vi "fgv buffer image references - measure tool.vi"(0 "Image Reference IN":T4, 1 "Actions":T1, 2 "Path":path, 5 "Imaging Parameters":T2, 9 "Calibration Parameters":T3, 11 "error in (no error)":errorcluster, 12 "index(s)":i32[](array[numeric]), 13 "element":string) -> (3 "Imag ref. name":string[](array[string]), 4 "Image Array":T4[](array[typedef]), 6 "LB data":string[][](array[string]), 8 "Imaging Parameters":T2[](array[typedef]), 10 "Calibration Parameters":T3[](array[typedef]), 14 "LB data full":string[][](array[string]), 15 "error out":errorcluster)   [LabVIEW 2020]
uses:
  <vilib>/vision/Image Controls.llb/IMAQ Image.ctl
  ToolBox/TypeDefs/Current Calibration Parameters.ctl
  ToolBox/TypeDefs/Current Imaging Parameters.ctl
  ToolBox/TypeDefs/data and image buffer fgv actions - measure tool.ctl
  138bf972-3e2c-4b9c-869a-8880fb0fa013.vi
  34bb193f-b545-427e-b1e4-c07e80b324ef.vi
  f5771faa-6821-441f-a328-0f121c78e6d9.vi
  d3480d6e-a209-486d-a997-ed0cab6325bc.vi
  <vilib>/Analysis/1siggen.llb/Ramp Pattern by Samples.vi
  <vilib>/Analysis/NI_AALBase.lvlib
panel:
  out "Sr No.":i32[](array[numeric])
  # "Note elements and index(s) are multi-use"
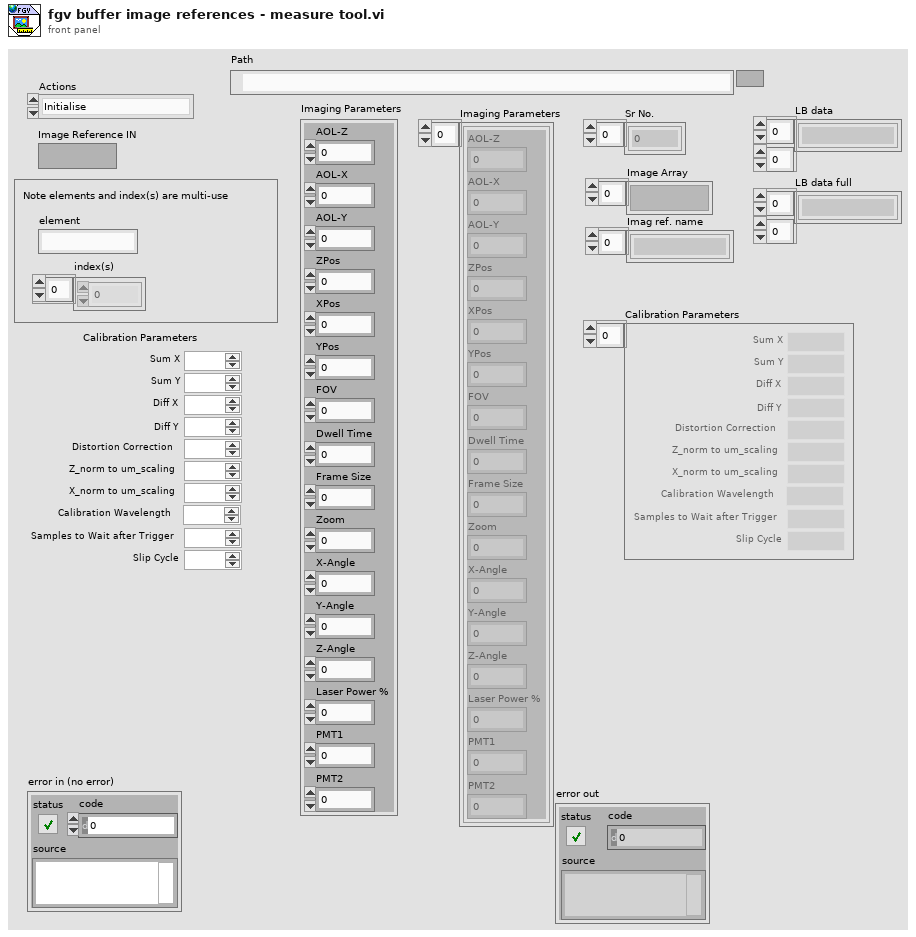
[diagram p1: front panel]
types:
  T1 = typedef "data and image buffer fgv actions - measure tool.ctl" = enum16{"Initialise", "Load Data from file", "Add Image to buffer", "Read Image buffer", "Edit specific data", "Delete selected image", "Clear all images"}
  T2 = typedef "Current Imaging Parameters.ctl" = cluster{"AOL-Z":dbl, "AOL-X":dbl, "AOL-Y":dbl, "ZPos":dbl, "XPos":dbl, "YPos":dbl, "FOV":dbl, "Dwell Time":dbl, "Frame Size":dbl, "Zoom":dbl, "X-Angle":dbl, "Y-Angle":dbl, "Z-Angle":dbl, "Laser Power %":dbl, "PMT1":dbl, "PMT2":dbl}
  T3 = typedef "Current Calibration Parameters.ctl" = cluster{"Sum X":dbl, "Sum Y":dbl, "Diff X":dbl, "Diff Y":dbl, "Distortion Correction":dbl, "Z_norm to um_scaling":dbl, "X_norm to um_scaling":dbl, "Samples to Wait after Trigger":dbl, "Slip Cycle":dbl, "Calibration Wavelength":dbl}
  T4 = typedef "IMAQ Image.ctl" = refnum<image>
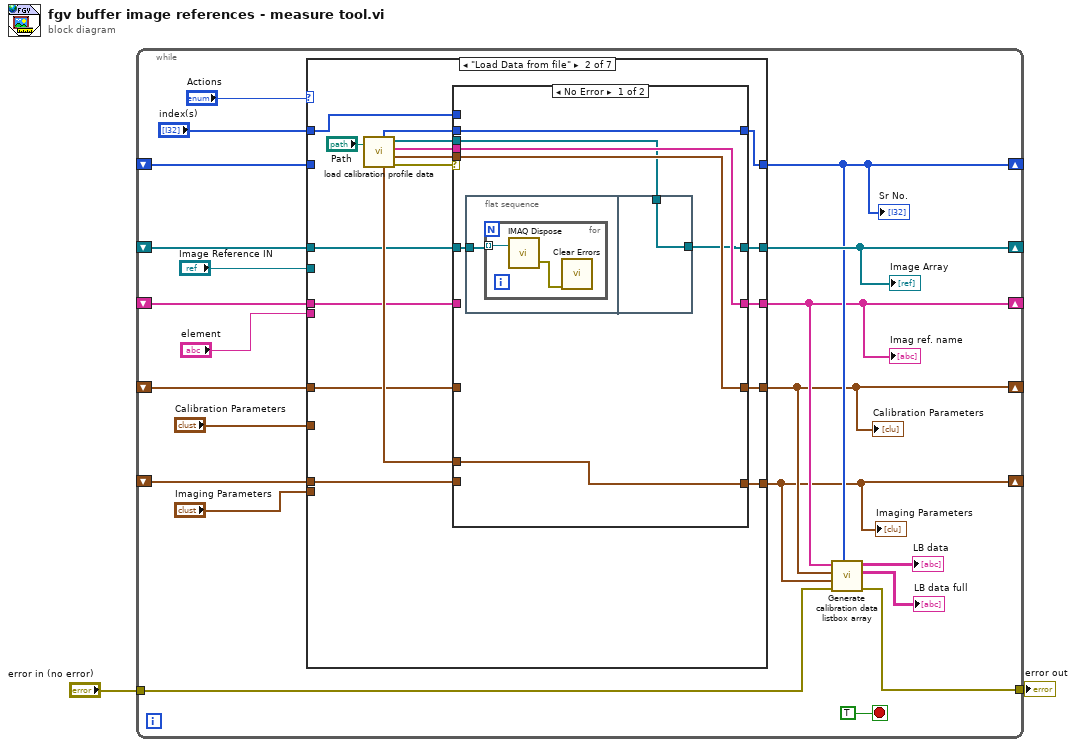
[diagram p0: block diagram]
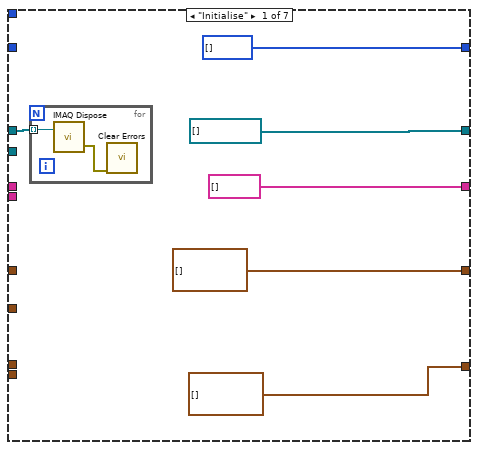
[diagram p2: hidden frame]
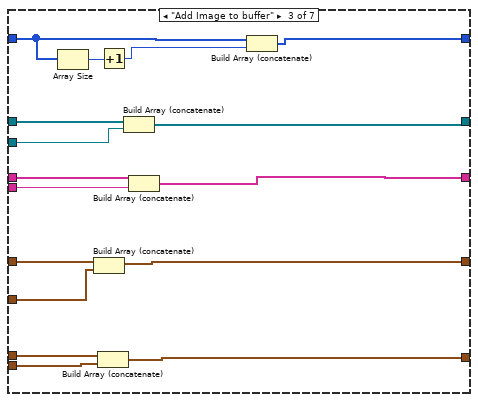
[diagram p4: hidden frame]
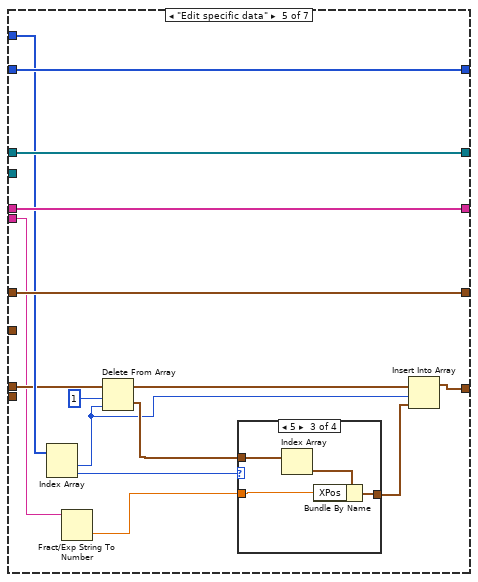
[diagram p6: hidden frame]
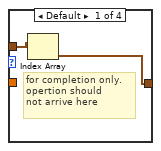
[diagram p7: hidden frame]
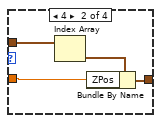
[diagram p8: hidden frame]
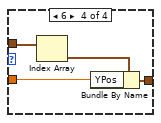
[diagram p9: hidden frame]
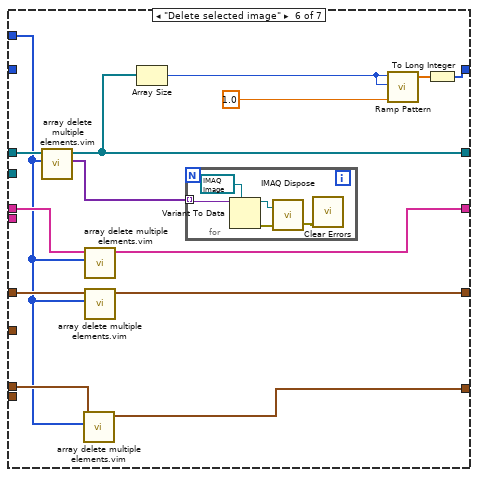
[diagram p10: hidden frame]
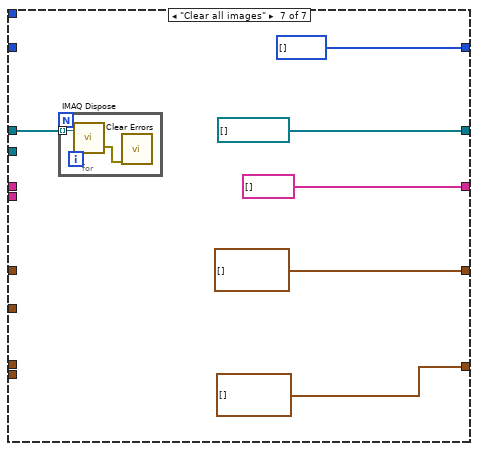
[diagram p11: hidden frame]
diagram:
  n1 = while {
    shift-right: [w22] -> _
    shift-left: _ -> [w21]
    tunnel: "error in (no error)" -> [w7]
    tunnel: [w6] -> w1
    shift-right: [w9] -> _
    shift-left: _ -> [w20]
    shift-right: [w8] -> _
    shift-left: _ -> [w18]
    shift-right: [w10] -> _
    shift-left: _ -> [w16]
    shift-right: [w11] -> _
    shift-left: _ -> [w12]
    stop <- TRUE stop-if-true
    n2 = case shown="\"Load Data from file\"" "Actions" {
      tunnel: [T4[] [] ("RedImageArray") w45 w79 w85 w99 w120 T4[] [] ("RedImageArray")] -> w22
      tunnel: w21 -> [w28 w35 w80 w85 w99 w124 w139]
      tunnel: "index(s)" -> [_ w37 _ _ w96 w116 _]
      tunnel: [T3[] [] w41 w65 w84 w97 w127 T3[] []] -> w9
      tunnel: w20 -> [_ w33 w78 w84 w97 w128 _]
      tunnel: "Calibration Parameters" -> [_ _ w77 _ _ _ _]
      tunnel: [T2[] [] w38 w67 w83 w86 w125 T2[] []] -> w8
      tunnel: w18 -> [_ w32 w76 w83 w95 w126 _]
      tunnel: "Imaging Parameters" -> [_ _ w75 _ _ _ _]
      tunnel: [string[] [] w43 w66 w81 w98 w115 string[] []] -> w10
      tunnel: w16 -> [_ w34 w74 w81 w98 w117 _]
      tunnel: "element" -> [_ _ w73 _ w91 _ _]
      tunnel: [i32[] [] w36 w68 w82 w100 w118 i32[] []] -> w11
      tunnel: "Image Reference IN" -> [_ _ w72 _ _ _ _]
      tunnel: w12 -> [_ _ w70 w82 w100 _ _]
      frame "Initialise" {
        n3 = for {
          tunnel: w28 -> [w31] mode=indexing
          n4 = call "IMAQ Dispose"("Image"=w31) -> ("error out"=w30:errorcluster)  [unwired: 5 in]
          n5 = call <vilib>:"Clear Errors.vi"("error in (no error)"=w30) -> ()  [unwired: 5 in, 2 out]
        }
      }
      frame "Load Data from file" {
        n6 = call "load calibration profile data.vi"("Path"="Path") -> ("error out"=w47:errorcluster, "Calibration params"=w40:T3[], "Image names"=w42:string[], "Image Array refs"=w44:T4[], "Scanning params"=w39:T2[], "Sr No."=w46:i32[])  [unwired: 5 in]
        n7 = case shown="No Error" w47 {
          tunnel: [w55 w64] -> w36
          tunnel: w46 -> [w55 _]
          tunnel: [w50 w63] -> w45
          tunnel: w44 -> [w49 _]
          tunnel: [w54 w62] -> w43
          tunnel: w42 -> [w54 _]
          tunnel: [w53 w61] -> w41
          tunnel: w40 -> [w53 _]
          tunnel: w39 -> [w52 _]
          tunnel: [w52 w60] -> w38
          tunnel: w37 -> [_ w64]
          tunnel: w35 -> [w51 w63]
          tunnel: w34 -> [_ w62]
          tunnel: w33 -> [_ w61]
          tunnel: w32 -> [_ w60]
          frame No Error {
            n8 = flat-sequence {
              tunnel: w51 -> [w56]
              tunnel: [w59] -> w50
              tunnel: w49 -> [w59]
              frame #0 {
                n9 = for {
                  tunnel: w56 -> [w58] mode=indexing
                  n10 = call "IMAQ Dispose"("Image"=w58) -> ("error out"=w57:errorcluster)  [unwired: 5 in]
                  n11 = call <vilib>:"Clear Errors.vi"("error in (no error)"=w57) -> ()  [unwired: 5 in, 2 out]
                }
              }
              frame #1 {
              }
            }
          }
          frame Error {
          }
        }
      }
      frame "Add Image to buffer" {
        n12 = Array Size(array=w70) -> (size(s)=w71:i32)
        n13 = Build Array (concatenate)(w78, w77) -> (w65:T3[])
        n14 = Build Array (concatenate)(w76, w75) -> (w67:T2[])
        n15 = Increment(x=w71) -> (x+1=w69:i32)
        n16 = Build Array (concatenate)(w80, w72) -> (w79:T4[])
        n17 = Build Array (concatenate)(w74, w73) -> (w66:string[])
        n18 = Build Array (concatenate)(w70, w69) -> (w68:i32[])
      }
      frame "Read Image buffer" {
      }
      frame "Edit specific data" {
        n19 = Index Array(array=w96) -> (element #1=w89:i32, element #2=w93:i32)  [unwired: 2 in]
        n20 = Fract/Exp String To Number(string=w91) -> (number=w90:dbl)  [unwired: 3 in, 1 out]
        n21 = Delete From Array(array=w95, length=1, index=w89) -> (deleted portion=w92:T2[], array with subset deleted=w88:T2[])
        n22 = case shown="5" w93 {
          tunnel: w92 -> [w102 w105 w109 w114]
          tunnel: w90 -> [_ w104 w108 w112]
          tunnel: [w101 w103 w107 w111] -> w87
          frame Default {
            # "for completion only.\nopertion should \nnot arrive here"
            n23 = Index Array(array=w102) -> (element=w101:T2)  [unwired: 1 in]
          }
          frame 4 {
            n24 = Index Array(array=w105) -> (element=w106:T2)  [unwired: 1 in]
            n25 = Bundle By Name(cluster=w106, "ZPos"=w104) -> (w103:T2)
          }
          frame 5 {
            n26 = Index Array(array=w109) -> (element=w110:T2)  [unwired: 1 in]
            n27 = Bundle By Name(cluster=w110, "XPos"=w108) -> (w107:T2)
          }
          frame 6 {
            n28 = Index Array(array=w114) -> (element=w113:T2)  [unwired: 1 in]
            n29 = Bundle By Name(cluster=w113, "YPos"=w112) -> (w111:T2)
          }
        }
        n30 = Insert Into Array(array=w88, index=w89, new element=w87) -> (w86:T2[])
      }
      frame "Delete selected image" {
        n31 = call "array delete multiple elements.vim"("Index(s)"=w116, "1D Array IN"=w124) -> ("Deleted Elemets"=w123:variant[], "1D Array OUT"=w120:T4[])  [unwired: 7 in, 1 out]
        n32 = call "array delete multiple elements.vim"("Index(s)"=w116, "1D Array IN"=w126) -> ("1D Array OUT"=w125:T2[])  [unwired: 7 in, 2 out]
        n33 = call "array delete multiple elements.vim"("Index(s)"=w116, "1D Array IN"=w117) -> ("1D Array OUT"=w115:string[])  [unwired: 7 in, 2 out]
        n34 = call "array delete multiple elements.vim"("Index(s)"=w116, "1D Array IN"=w128) -> ("1D Array OUT"=w127:T3[])  [unwired: 7 in, 2 out]
        n35 = Array Size(array=w120) -> (size(s)=w119:i32)
        n36 = for {
          tunnel: w123 -> [w133] mode=indexing
          n37 = Variant To Data(type=T4 refnum ("Image"), Variant=w133) -> (data=w131:T4, error out=w130:errorcluster)  [unwired: 1 in]
          n38 = call "IMAQ Dispose"("Image"=w131, "error in (no error)"=w130) -> ("error out"=w129:errorcluster)  [unwired: 4 in]
          n39 = call <vilib>:"Clear Errors.vi"("error in (no error)"=w129) -> ()  [unwired: 5 in, 2 out]
        }
        n40 = call-poly <vilib>:"Ramp Pattern.vi"("start"=1.0, "end"=w119, "samples"=w119) -> ("Ramp Pattern"=w121:dbl[])  [unwired: 7 in, 1 out]
        n41 = To Long Integer(number=w121) -> (32bit integer=w118:i32[])
      }
      frame "Clear all images" {
        n42 = for {
          tunnel: w139 -> [w141] mode=indexing
          n43 = call "IMAQ Dispose"("Image"=w141) -> ("error out"=w140:errorcluster)  [unwired: 5 in]
          n44 = call <vilib>:"Clear Errors.vi"("error in (no error)"=w140) -> ()  [unwired: 5 in, 2 out]
        }
      }
    }
    "Image Array" <- w22
    "Calibration Parameters" <- w9
    "Imaging Parameters" <- w8
    "Imag ref. name" <- w10
    "Sr No." <- w11
    n45 = call "Generate calibration data listbox array .vi"("Sr No."=w11, "error in (no error)"=w7, "Imaging Parameters"=w8, "Calibration data"=w9, "Imag ref. name"=w10) -> ("error out"=w6:errorcluster, "LB data full"=→"LB data full":string[][], "LB data trunc"=→"LB data":string[][])  [unwired: 4 in]
  }
  "error out" <- w1
